vi "Popup - Login Screen.vi"(8 "error in (no error)":errorcluster, 11 "Controller (Host) Data in":T2={"Instr Initialized?"=FALSE, "State"=enum."APU Select", "APU Select"="<Select>", "Testing Type Select"=enum."Manual", "Login Info"={"Username"="", "Login Access"=enum."Admin"}, "2D User Info"=[], "APU Setup File"={"[[Sensor Info]]"=[], "[[Calibration Info]]"=[], "[[CMM Table 106]]"=[], "[[General APU Info]]"=[], "General APU Information"={"Run Count"=0}, "[[CMM Table 106B]] "=[]}, "Test Information"={"APU Part Number:"="", "Model:"="", "Serial Number:"="", "Customer:"="", "Work Order:"="", "Repair Level:"=""}, "Report Filepath"=path "", "Run Count increase Available? "=FALSE, "SubTest"="", "Numeric Control"=0.0}) -> (0 "error out":errorcluster, 2 "Login Info":cluster{"Username":string, "Login Access":T1}, 3 "Controller (Host) Data out":T2={"Instr Initialized?"=FALSE, "State"=enum."APU Select", "APU Select"="<Select>", "Testing Type Select"=enum."Manual", "Login Info"={"Username"="", "Login Access"=enum."Admin"}, "2D User Info"=[], "APU Setup File"={"[[Sensor Info]]"=[], "[[Calibration Info]]"=[], "[[CMM Table 106]]"=[], "[[General APU Info]]"=[], "General APU Information"={"Run Count"=0}, "[[CMM Table 106B]] "=[]}, "Test Information"={"APU Part Number:"="", "Model:"="", "Serial Number:"="", "Customer:"="", "Work Order:"="", "Repair Level:"=""}, "Report Filepath"=path "", "Run Count increase Available? "=FALSE, "SubTest"="", "Numeric Control"=0.0}, 4 "Exit?":bool)   [LabVIEW 2018]
doc: "This is the login dialog."
uses:
  Private Controls/Controller (Host) Data.ctl
  Private Controls/State.ctl
  Public Controls/APU Select.ctl
  Public Controls/Testing Select.ctl
  Public Controls/Login Access.ctl
  Top Level/Shared Controls/APU Setup File.ctl
  File IO/Public Controls/General APU Info.ctl
  Public Controls/Test Information.ctl
  Controller (Host).lvlib
  File IO/File IO.lvlib
panel:
  in  "Submit":bool
  in  "Guest Login":bool
  in  "Password":string="Password"
  in  "Username":string="Username"
  in  "Exit":bool
  # "Login"
  # "Test Information:"
  # "Test Information:"
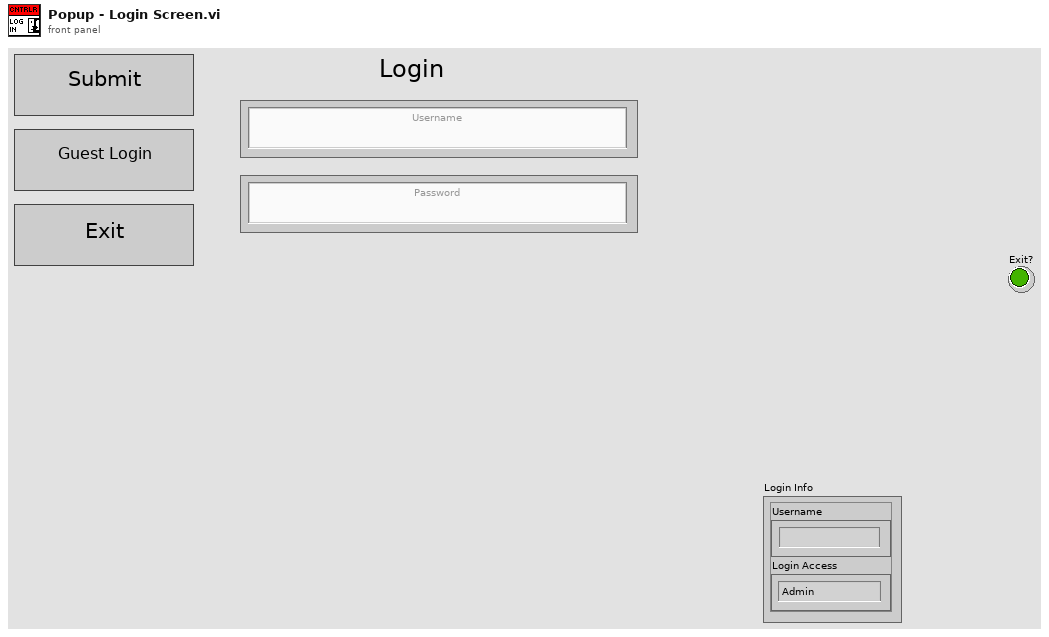
[diagram p1: front panel]
types:
  T1 = typedef "Controller (Host).lvlib/Login Access.ctl" = enum16{"Admin", "Operator", "Guest", ""}
  T2 = typedef "Controller (Host).lvlib/Controller (Host) Data.ctl" = cluster{"Instr Initialized?":bool, "State":T3, "APU Select":T4, "Testing Type Select":T5, "Login Info":cluster{"Username":string, "Login Access":T1}, "2D User Info":string[][], "APU Setup File":T6, "Test Information":T8, "Report Filepath":path, "Run Count increase Available? ":bool, "SubTest":string, "Numeric Control":dbl}
  T3 = typedef "Controller (Host).lvlib/State.ctl" = enum16{"APU Select", "Operation Select", "SubTests Select", "Calibration", "Testing", "Exit"}
  T4 = typedef "Controller (Host).lvlib/APU Select.ctl" = string
  T5 = typedef "Controller (Host).lvlib/Testing Select.ctl" = enum16{"Manual", "Interactive", "Automatic"}
  T6 = typedef "APU Setup File.ctl" = cluster{"[[Sensor Info]]":string[][], "[[Calibration Info]]":string[][], "[[CMM Table 106]]":string[][], "[[General APU Info]]":string[][], "General APU Information":T7, "[[CMM Table 106B]] ":string[][]}
  T7 = typedef "File IO.lvlib/General APU Info.ctl" = cluster{"Run Count":u64}
  T8 = typedef "Controller (Host).lvlib/Test Information.ctl" = cluster{"APU Part Number:":string, "Model:":string, "Serial Number:":string, "Customer:":string, "Work Order:":string, "Repair Level:":string}
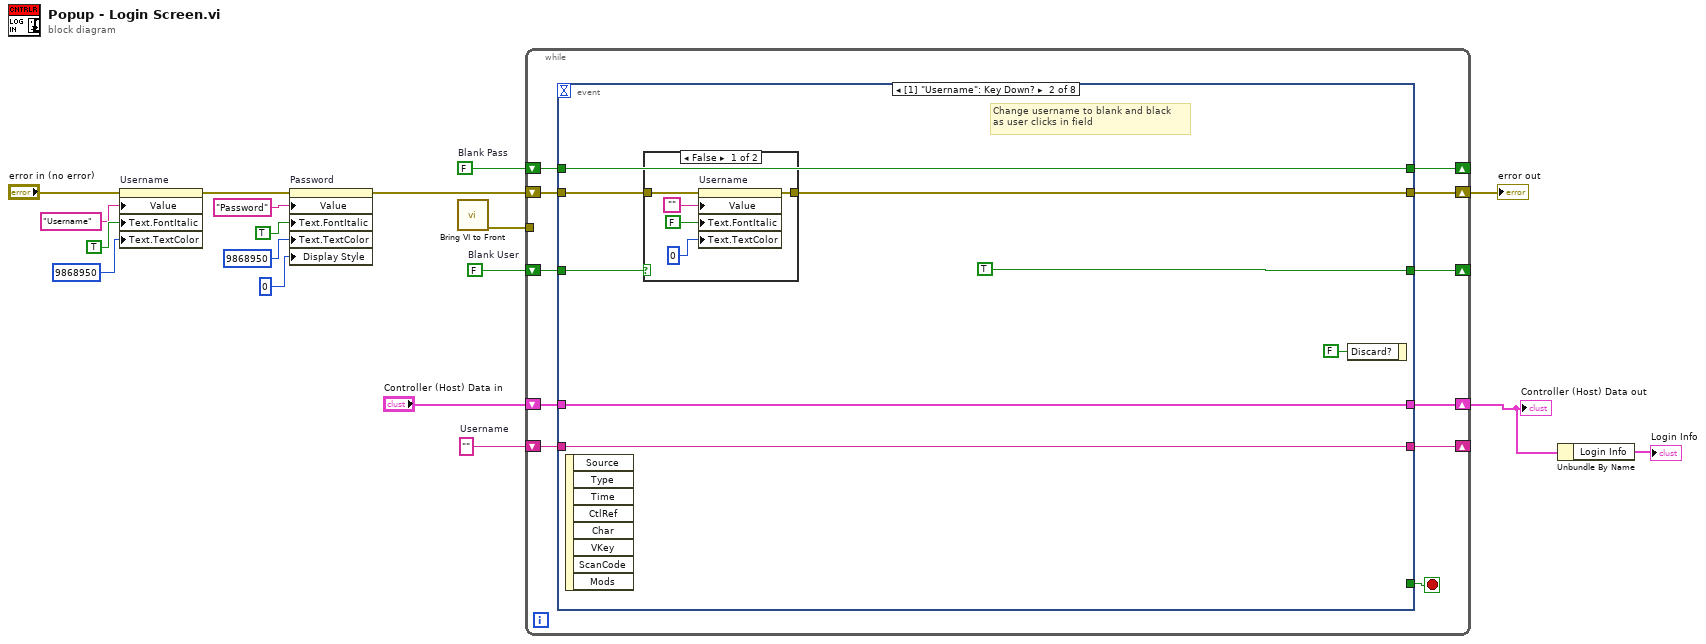
[diagram p0: block diagram]
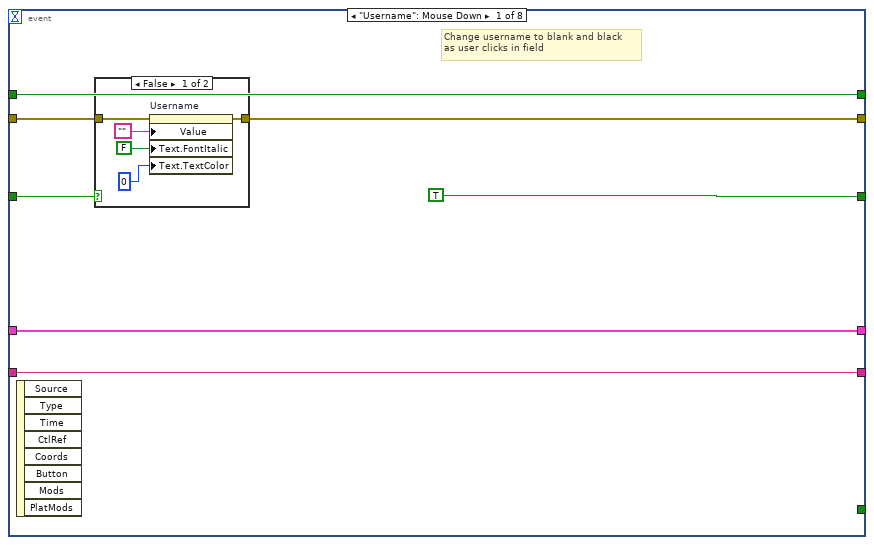
[diagram p2: hidden frame]
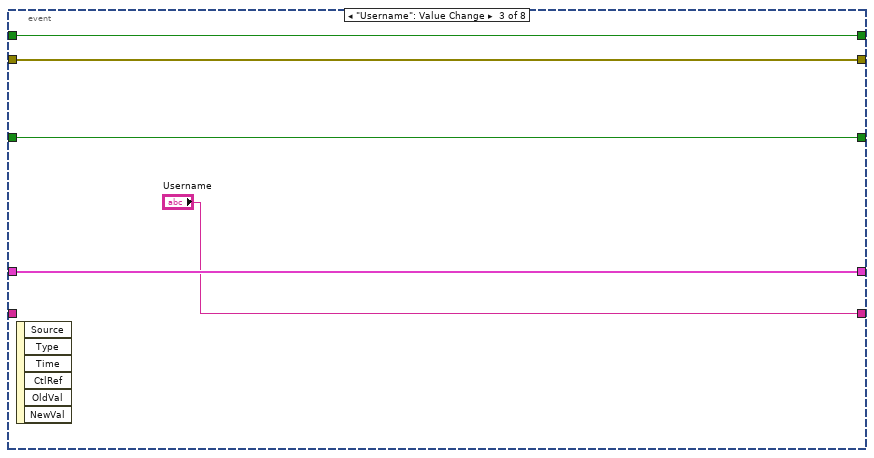
[diagram p5: hidden frame]
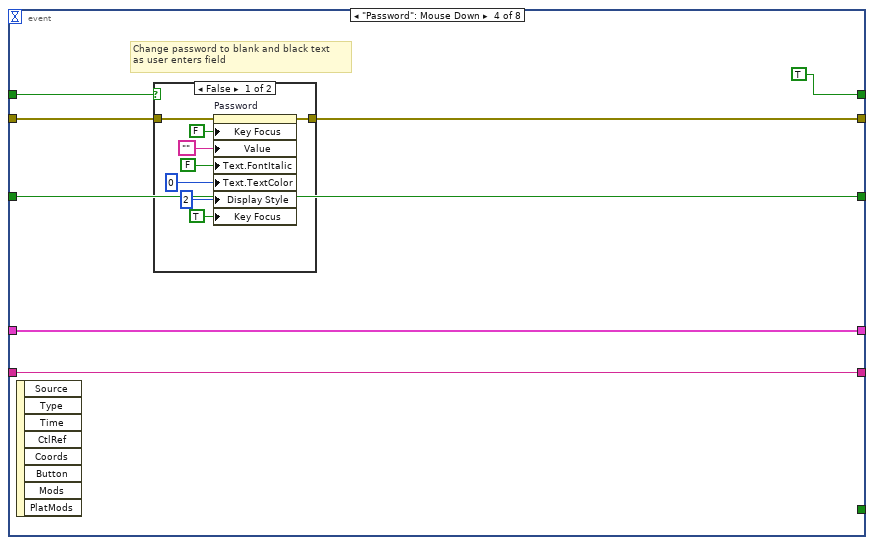
[diagram p6: hidden frame]
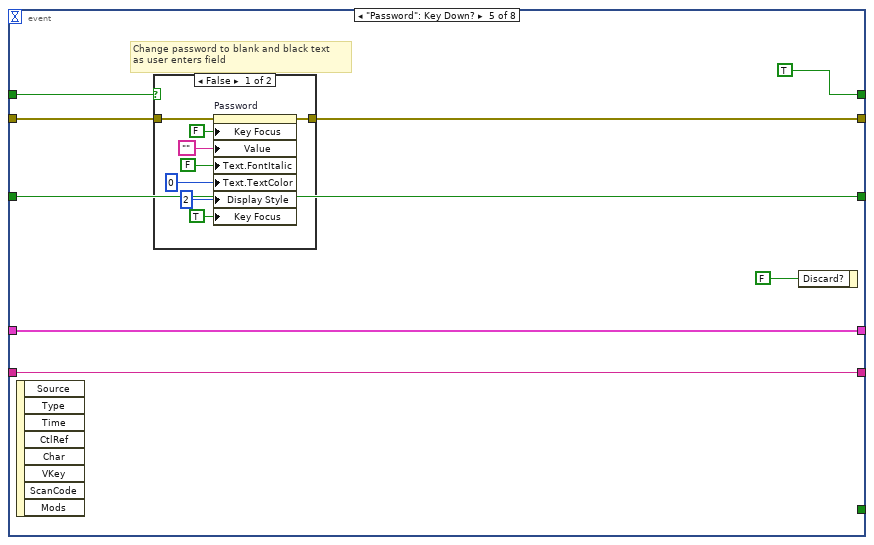
[diagram p8: hidden frame]
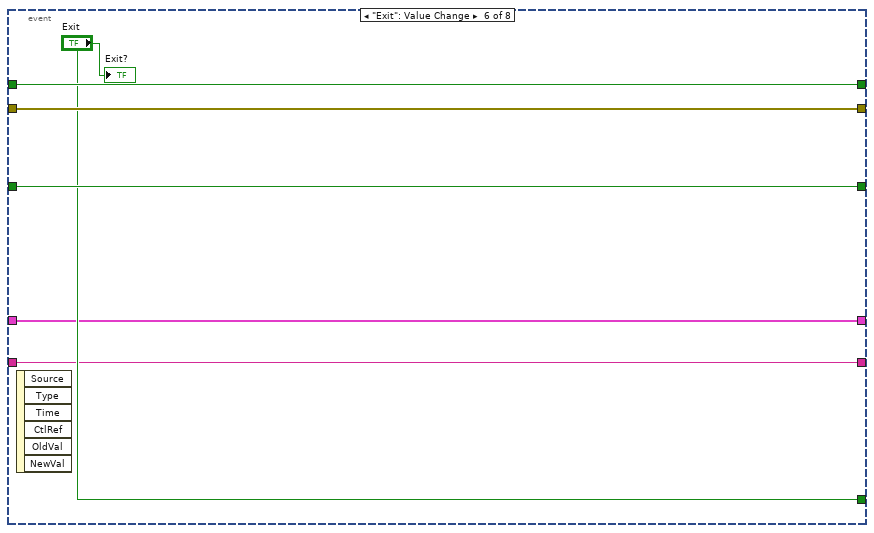
[diagram p10: hidden frame]
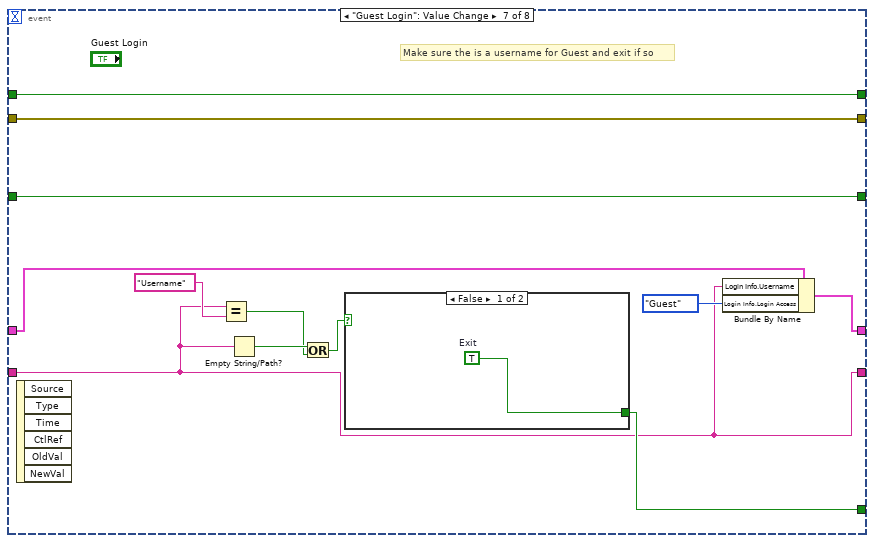
[diagram p11: hidden frame]
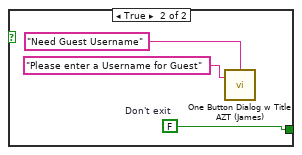
[diagram p12: hidden frame]
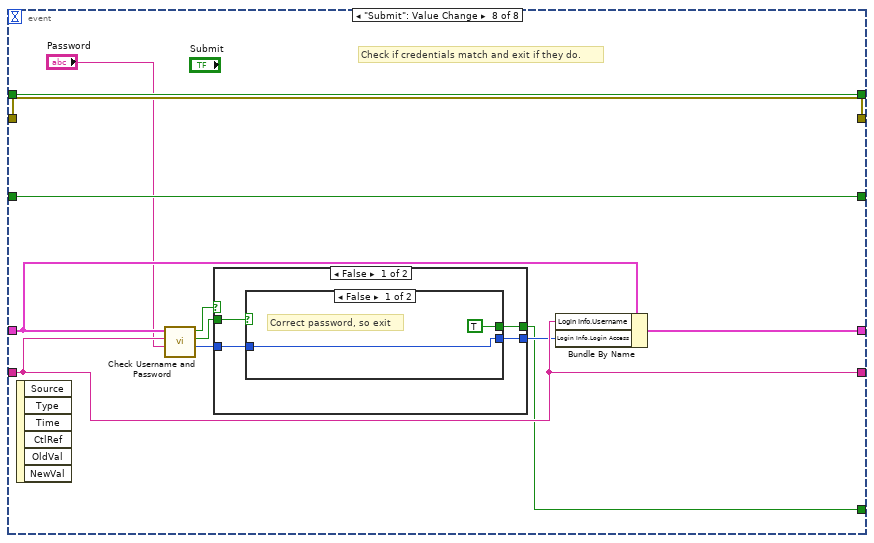
[diagram p13: hidden frame]
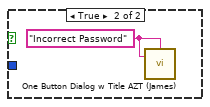
[diagram p14: hidden frame]
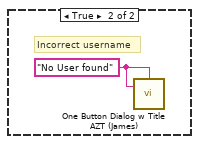
[diagram p15: hidden frame]
diagram:
  w4 = ""  # Username
  w11 = FALSE  # Blank Pass
  w10 = FALSE  # Blank User
  n1 = property on="Username" class="Str"(error in="error in (no error)", "Value"="Username" ("Username"), "Text.FontItalic"=TRUE ("Text.Font:Italic"), "Text.TextColor"=u32 9868950 ("Text.Text Colors:Text Color")) -> (error out=w13:errorcluster)  [unwired: 1 in, 1 out]
  n2 = property on="Password" class="Str"(error in=w13, "Value"="Password" ("Username"), "Text.FontItalic"=TRUE ("Text.Font:Italic"), "Text.TextColor"=u32 9868950 ("Text.Text Colors:Text Color"), "Display Style"=u32 0) -> (error out=w12:errorcluster)  [unwired: 1 in, 1 out]
  n3 = call "Bring VI to Front.vi"() -> ("error out"=w1:errorcluster)  [unwired: 11 in]
  n4 = while {
    shift-right: [w26] -> _
    shift-left: w11 -> [w28]
    shift-right: [w27] -> _
    shift-left: w10 -> [w29]
    shift-right: [w24] -> w5
    shift-left: w12 -> [w25]
    shift-right: [w21] -> w3
    shift-left: "Controller (Host) Data in" -> [w22]
    shift-right: [w20] -> _
    shift-left: w4 -> [w19]
    tunnel: w1 -> [_]
    stop <- w23 stop-if-true
    n5 = event shown="[1] \"Username\": Key Down?" {
      selector: _ -> [_ _ _ _ _ _ _ _]
      dyn-events: _ -> [_ _ _ _ _ _ _ _]
      timeout: _ -> [_ _ _ _ _ _ _ _]
      tunnel: w29 -> [w36 w50 w61 w63 w80 w100 w112 w128]
      tunnel: w28 -> [w35 w49 w60 w65 w82 w99 w111 w127]
      tunnel: [TRUE TRUE w61 w63 w80 w100 w112 w128] -> w27
      tunnel: [w35 w49 w60 TRUE ("Blank Pass") TRUE ("Blank Pass") w99 w111 w127] -> w26
      tunnel: w25 -> [w32 w46 w59 w68 w85 w98 w110 w126]
      tunnel: [w33 w47 w59 w67 w84 w98 w110 w126] -> w24
      tunnel: [_ _ _ _ _ "Exit" w106 w117] -> w23
      tunnel: w22 -> [w31 w45 w58 w66 w83 w96 w109 w124]
      tunnel: [w31 w45 w58 w66 w83 w96 w108 w125] -> w21
      tunnel: w19 -> [w30 w44 _ w62 w79 w95 w101 w123]
      tunnel: [w30 w44 "Username" w62 w79 w95 w101 w123] -> w20
      event "Username": Mouse Down {
        # "Change username to blank and black\nas user clicks in field"
        n6 = event-data() -> ()  [unwired: 1 in, 8 out]
        n7 = case shown="False" w36 {
          tunnel: [w37 w42] -> w33
          tunnel: w32 -> [w38 w42]
          frame False {
            n8 = property on="Username" class="Str"(error in=w38, "Value"="", "Text.FontItalic"=FALSE ("Text.Font:Italic"), "Text.TextColor"=u32 0 ("Text.Text Colors:Text Color")) -> (error out=w37:errorcluster)  [unwired: 1 in, 1 out]
          }
          frame True {
          }
        }
      }
      event "Username": Key Down? {
        # "Change username to blank and black\nas user clicks in field"
        n9 = event-data() -> ()  [unwired: 1 in, 8 out]
        n10 = case shown="False" w50 {
          tunnel: [w51 w56] -> w47
          tunnel: w46 -> [w52 w56]
          frame False {
            n11 = property on="Username" class="Str"(error in=w52, "Value"="", "Text.FontItalic"=FALSE ("Text.Font:Italic"), "Text.TextColor"=u32 0 ("Text.Text Colors:Text Color")) -> (error out=w51:errorcluster)  [unwired: 1 in, 1 out]
          }
          frame True {
          }
        }
        n12 = event-data("Discard?"=FALSE) -> ()  [unwired: 1 in, 1 out]
      }
      event "Username": Value Change {
        n13 = event-data() -> ()  [unwired: 1 in, 6 out]
      }
      event "Password": Mouse Down {
        # "Change password to blank and black text\nas user enters field"
        n14 = event-data() -> ()  [unwired: 1 in, 8 out]
        n15 = case shown="False" w65 {
          tunnel: w68 -> [w73 w77]
          tunnel: [w72 w77] -> w67
          frame False {
            n16 = property on="Password" class="Str"(error in=w73, "Key Focus"=FALSE, "Value"="", "Text.FontItalic"=FALSE ("Text.Font:Italic"), "Text.TextColor"=u32 0 ("Text.Text Colors:Text Color"), "Display Style"=u32 2, "Key Focus"=TRUE) -> (error out=w72:errorcluster)  [unwired: 1 in, 1 out]
          }
          frame True {
          }
        }
      }
      event "Password": Key Down? {
        # "Change password to blank and black text\nas user enters field"
        n17 = event-data() -> ()  [unwired: 1 in, 8 out]
        n18 = case shown="False" w82 {
          tunnel: w85 -> [w90 w94]
          tunnel: [w89 w94] -> w84
          frame False {
            n19 = property on="Password" class="Str"(error in=w90, "Key Focus"=FALSE, "Value"="", "Text.FontItalic"=FALSE ("Text.Font:Italic"), "Text.TextColor"=u32 0 ("Text.Text Colors:Text Color"), "Display Style"=u32 2, "Key Focus"=TRUE) -> (error out=w89:errorcluster)  [unwired: 1 in, 1 out]
          }
          frame True {
          }
        }
        n20 = event-data("Discard?"=FALSE) -> ()  [unwired: 1 in, 1 out]
      }
      event "Exit": Value Change {
        n21 = event-data() -> ()  [unwired: 1 in, 6 out]
        "Exit?" <- "Exit"
      }
      event "Guest Login": Value Change {
        # "Make sure the is a username for Guest and exit if so"
        n22 = event-data() -> ()  [unwired: 1 in, 6 out]
        n23 = Equal?(x=w101, y="Username") -> (x = y?=w102:bool)
        n24 = Empty String/Path?(string/path=w101) -> (empty?=w104:bool)
        n25 = Or(x=w104, y=w102) -> (x .or. y?=w105:bool)
        n26 = case shown="False" w105 {
          tunnel: [w113 w116] -> w106
          frame False {
            w113 = TRUE  # Exit
          }
          frame True {
            w116 = FALSE  # Don't exit
            n27 = call "One Button Dialog w Title AZT (James).vi"("Window Title (\"\")"="Need Guest Username" ("Window Title (\"\")"), "message"="Please enter a Username for Guest") -> ()  [unwired: 1 in, 1 out]
          }
        }
        n28 = Bundle By Name(cluster=w109, "Login Info.Username"=w101, "Login Info.Login Access"=Login_Access."Guest") -> (w108:T2)
      }
      event "Submit": Value Change {
        # "Check if credentials match and exit if they do."
        n29 = event-data() -> ()  [unwired: 1 in, 6 out]
        n30 = call "Check Username and Password.vi"("Password"="Password", "Username"=w123, "Controller (Host) Data in"=w124) -> ("Access"=w118:i32, "Incorrect Password"=w119:bool, "Incorrect username"=w121:bool)  [unwired: 6 in]
        n31 = case shown="False" w121 {
          tunnel: [w131 _] -> w117
          tunnel: [w130 _] -> w120
          tunnel: w119 -> [w132 _]
          tunnel: w118 -> [w129 _]
          frame False {
            n32 = case shown="False" w132 {
              tunnel: [TRUE ("true") _] -> w131
              tunnel: [w134 _] -> w130
              tunnel: w129 -> [w134 _]
              frame False {
                # "Correct password, so exit"
              }
              frame True {
                w135 = "Incorrect Password" ("message")
                n33 = call "One Button Dialog w Title AZT (James).vi"("Window Title (\"\")"=w135, "message"=w135) -> ()  [unwired: 1 in, 1 out]
              }
            }
          }
          frame True {
            w136 = "No User found" ("message")
            # "Incorrect username"
            n34 = call "One Button Dialog w Title AZT (James).vi"("Window Title (\"\")"=w136, "message"=w136) -> ()  [unwired: 1 in, 1 out]
          }
        }
        n35 = Bundle By Name(cluster=w124, "Login Info.Username"=w123, "Login Info.Login Access"=w120) -> (w125:T2)
      }
    }
  }
  "error out" <- w5
  "Controller (Host) Data out" <- w3
  n36 = Unbundle By Name(w3) -> ("Login Info"=→"Login Info":cluster{"Username":string, "Login Access":T1})
